vi "Communicate Stream Read.vi"(8 "error in":errorcluster, 11 "Call ID in":T2) -> (0 "error out":errorcluster, 1 "Success":bool, 2 "Response Data":T1, 3 "Call ID":T2)   [LabVIEW 2021, in "Demo_client.lvlib"]
uses:
  Demo_client.lvlib
  <vilib>/gRPC/LabVIEW gRPC Library/Shared/grpcId.ctl
  RPC Messages/Communication_StreamData.ctl
  aea5dbbb-03a2-479b-ad95-94da4ee1cea9.vi
  <vilib>/gRPC/LabVIEW gRPC Library/Shared/TranslateGrpcError.vi
  <vilib>/gRPC/LabVIEW gRPC Library/Shared/Wait On Occurence.vi
  <vilib>/gRPC/LabVIEW gRPC Library/Server API/Server/Get Server DLL Path.vi
  <vilib>/Utility/error.llb/Error Cluster From Error Code.vi
  <vilib>/Utility/error.llb/Simple Error Handler.vi
  <vilib>/gRPC/LabVIEW gRPC Library/grpc-lvsupport-release.lvlib
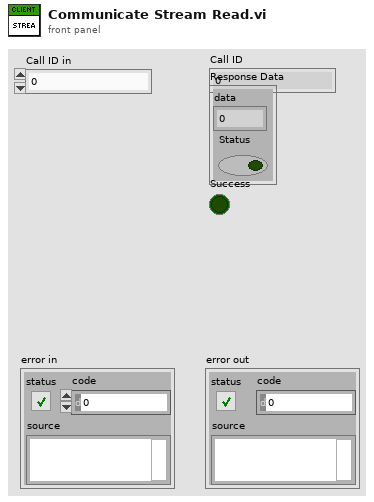
[diagram p1: front panel]
types:
  T1 = typedef "Demo_client.lvlib/Communication_StreamData.ctl" = cluster{"data":i32, "Status":bool}
  T2 = typedef "grpc-lvsupport-release.lvlib/grpcId.ctl" = u64
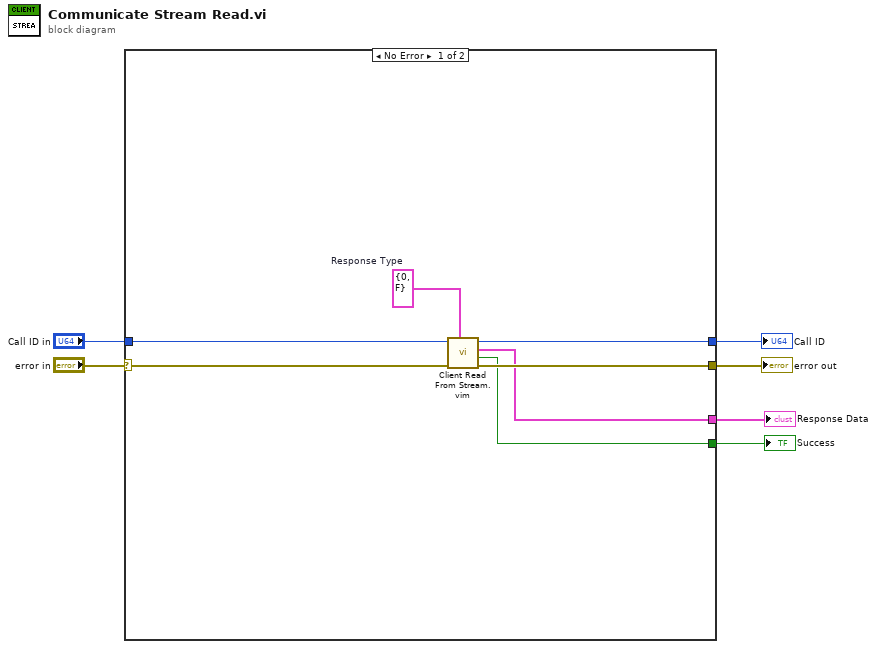
[diagram p0: block diagram]
diagram:
  n1 = case shown="No Error" "error in" {
    selector: "error in" -> [w13 w14]
    tunnel: [w12 w14] -> w5
    tunnel: "Call ID in" -> [w11 w15]
    tunnel: [w7 w15] -> w3
    tunnel: [w10 _] -> w2
    tunnel: [w8 _] -> w1
    frame No Error {
      w9 = T1 {"data"=0, "Status"=FALSE}  # Response Type
      n2 = call "Client Read From Stream.vim"("Response Type"=w9, "error in"=w13, "Call ID in"=w11) -> ("error out"=w12:errorcluster, "Success"=w8:bool, "Response Data"=w10:T1, "Call ID out"=w7:u64)  [unwired: 5 in]
    }
    frame Error {
    }
  }
  "error out" <- w5
  "Call ID" <- w3
  "Response Data" <- w2
  "Success" <- w1
